vi "Bar to meter.vi"(9 "g":dbl format="%#_13g", 10 "H [bar]":dbl, 11 "Dens":dbl) -> (2 "H[m]":dbl)   [LabVIEW 2019]
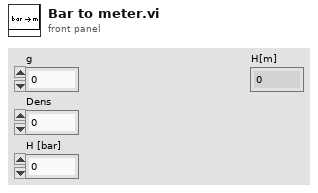
[diagram p1: front panel]
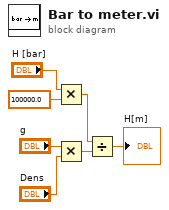
[diagram p0: block diagram]
diagram:
  n1 = Multiply(x="H [bar]", y=100000.0) -> (x*y=w4:dbl)
  n2 = Multiply(x="g", y="Dens") -> (x*y=w5:dbl)
  n3 = Divide(x=w4, y=w5) -> (x/y=→"H[m]":dbl)
